vi "KonfigLesen.vi"(1 "Dateipfad (Dialog verwenden)":path) -> (0 "MethodenNamen":string[](array[string]))   [LabVIEW 2010]
uses:
  <vilib>/regexp/Match Regular Expression.xnode
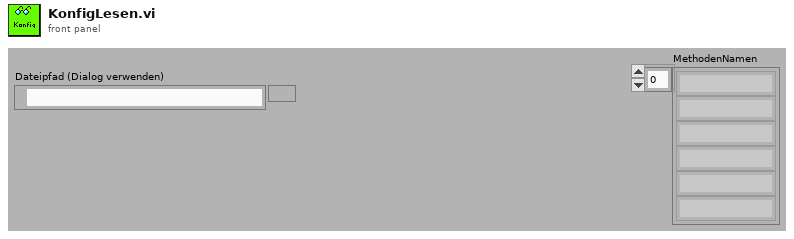
[diagram p1: front panel]
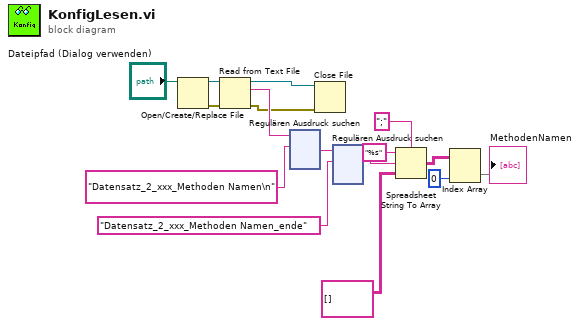
[diagram p0: block diagram]
diagram:
  n1 = Open/Create/Replace File(file path (use dialog)="Dateipfad (Dialog verwenden)") -> (refnum out=w14:refnum<file>, error out=w15:errorcluster)  [unwired: 5 in, 1 out]
  n2 = Read from Text File(file (use dialog)=w14, error in=w15) -> (refnum out=w5:refnum<file>, text=w13:string, error out=w4:errorcluster)  [unwired: 2 in, 1 out]
  n3 = xnode "Regulären Ausdruck suchen"("Eingangs-String"=w13, "Regulärer Ausdruck"="Datensatz_2_xxx_Methoden Namen\n") -> ("Nach Übereinstimmung"=w11:string)  [unwired: 4 in, 4 out]
  n4 = Close File(refnum=w5, error in=w4) -> ()  [unwired: 2 out]
  n5 = xnode "Regulären Ausdruck suchen"("Eingangs-String"=w11, "Regulärer Ausdruck"="Datensatz_2_xxx_Methoden Namen_ende") -> ("Vor Übereinstimmung"=w9:string)  [unwired: 4 in, 4 out]
  n6 = Spreadsheet String To Array(delimiter (Tab)=";" ("Trennzeichen (Tabulator)"), format string="%s" ("Format-String"), spreadsheet string=w9, array type (2D Dbl)=string[][] []) -> (array=w3:string[][])
  n7 = Index Array(array=w3, index (col)=0 ("Deaktivierter Index (Spalte)")) -> (element=→"MethodenNamen":string[])  [unwired: 1 in]
